vi "triggerIRQInstructionFA.vi"(8 "error in (no error)":errorcluster, 10 "ModbusBuffer in":refnum<class "ModbusBuffer.lvclass">, 11 "ILCCommunications in":refnum<class "ILCCommunications.lvclass">) -> (0 "error out":errorcluster, 2 "ModbusBuffer out":refnum<class "ModbusBuffer.lvclass">, 3 "ILCCommunications out":refnum<class "ILCCommunications.lvclass">)   [LabVIEW 2016, in "ILCCommunications.lvclass"]
uses:
  ILCCommunications.lvclass
  Common_RT_Modbus/ModbusBuffer/ModbusBuffer.lvclass
  Common_RT_Modbus/ModbusBuffer/ModbusBuffer.lvclass/ModbusBuffer.ctl
  Common_RT_Modbus/ModbusBuffer/writeTriggerIRQ.vi
  Common_RT_Modbus/ModbusBuffer/writeHeader.vi
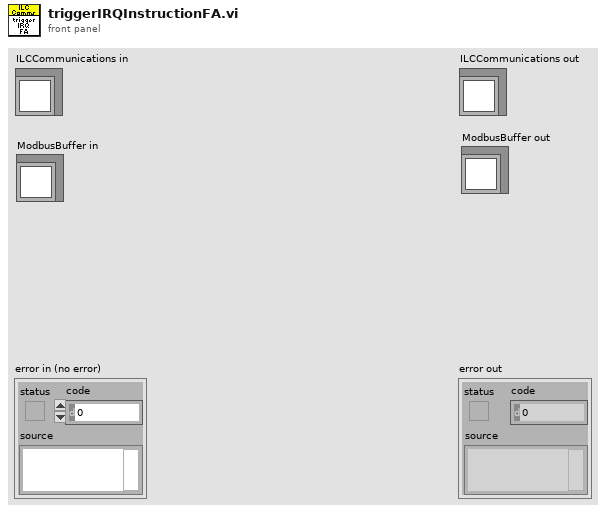
[diagram p1: front panel]
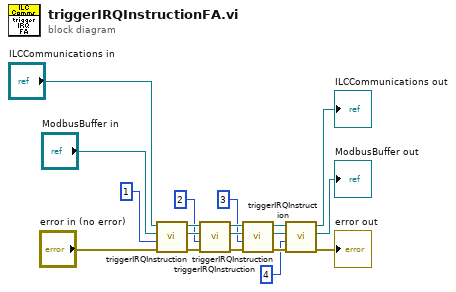
[diagram p0: block diagram]
diagram:
  n1 = call "triggerIRQInstruction.vi"("error in (no error)"="error in (no error)", "Subnet"=u8 1, "ModbusBuffer in"="ModbusBuffer in", "ILCCommunications in"="ILCCommunications in") -> ("error out"=w15:errorcluster, "ModbusBuffer out"=w14:refnum<class "ModbusBuffer.lvclass">, "ILCCommunications out"=w13:refnum<class "ILCCommunications.lvclass">)  [unwired: 5 in]
  n2 = call "triggerIRQInstruction.vi"("error in (no error)"=w15, "Subnet"=u8 2, "ModbusBuffer in"=w14, "ILCCommunications in"=w13) -> ("error out"=w12:errorcluster, "ModbusBuffer out"=w11:refnum<class "ModbusBuffer.lvclass">, "ILCCommunications out"=w10:refnum<class "ILCCommunications.lvclass">)  [unwired: 5 in]
  n3 = call "triggerIRQInstruction.vi"("error in (no error)"=w12, "Subnet"=u8 3, "ModbusBuffer in"=w11, "ILCCommunications in"=w10) -> ("error out"=w9:errorcluster, "ModbusBuffer out"=w8:refnum<class "ModbusBuffer.lvclass">, "ILCCommunications out"=w7:refnum<class "ILCCommunications.lvclass">)  [unwired: 5 in]
  n4 = call "triggerIRQInstruction.vi"("error in (no error)"=w9, "Subnet"=u8 4, "ModbusBuffer in"=w8, "ILCCommunications in"=w7) -> ("error out"=→"error out":errorcluster, "ModbusBuffer out"=→"ModbusBuffer out":refnum<class "ModbusBuffer.lvclass">, "ILCCommunications out"=→"ILCCommunications out":refnum<class "ILCCommunications.lvclass">)  [unwired: 5 in]
